vi "Construct Message.vi"(3 "Data":variant, 4 "Command":string, 5 "Destination":string, 6 "Source":string) -> (0 "output cluster":T1={"Source"="", "Destination"="", "Time Stamp"=timestamp(0 s since 1904-01-01), "Command"="", "Data"=variant(string "")})   [LabVIEW 2020, in "Dynamic Reentrant.lvlib"]
uses:
  <userlib>/Dynamic Reentrant/Dynamic Reentrant.lvlib
  <userlib>/Dynamic Reentrant/Type Defs/Message.ctl
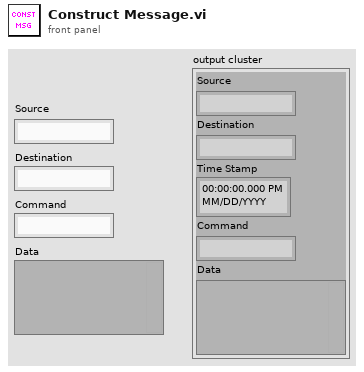
[diagram p1: front panel]
types:
  T1 = typedef "Dynamic Reentrant.lvlib/Message.ctl" = cluster{"Source":string, "Destination":string, "Time Stamp":timestamp, "Command":string, "Data":variant}
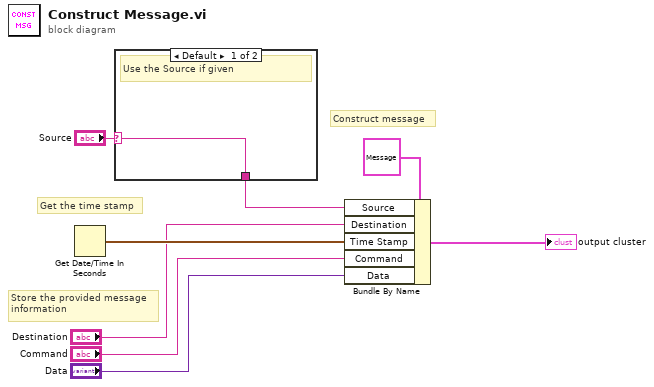
[diagram p0: block diagram]
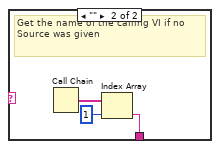
[diagram p2: hidden frame]
diagram:
  # "Construct message"
  # "Store the provided message\ninformation"
  # "Get the time stamp"
  n1 = Get Date/Time In Seconds() -> (seconds since 1Jan1904=w5:timestamp)
  n2 = case shown="Default" "Source" {
    selector: "Source" -> [w9 _]
    tunnel: [w9 w10] -> w1
    frame Default {
      # "Use the Source if given"
    }
    frame "" {
      # "Get the name of the calling VI if no Source was given"
      n3 = Call Chain() -> (call chain=w12:string[])
      n4 = Index Array(array=w12, index=1) -> (element=w10:string)
    }
  }
  n5 = Bundle By Name(cluster=T1 {"Source"="", "Destination"="", "Time Stamp"=timestamp(0 s since 1904-01-01), "Command"="", "Data"=variant(string "")} ("Message"), "Source"=w1, "Destination"="Destination", "Time Stamp"=w5, "Command"="Command", "Data"="Data") -> (→"output cluster":T1)
